vi "Move LabVIEW File.vi"(8 "error in (no error)":errorcluster, 10 "New Path":path, 11 "Existing Path":path) -> (0 "error out":errorcluster)   [LabVIEW 2016, in "SLL Scripting.lvlib"]
uses:
  SLL Scripting.lvlib
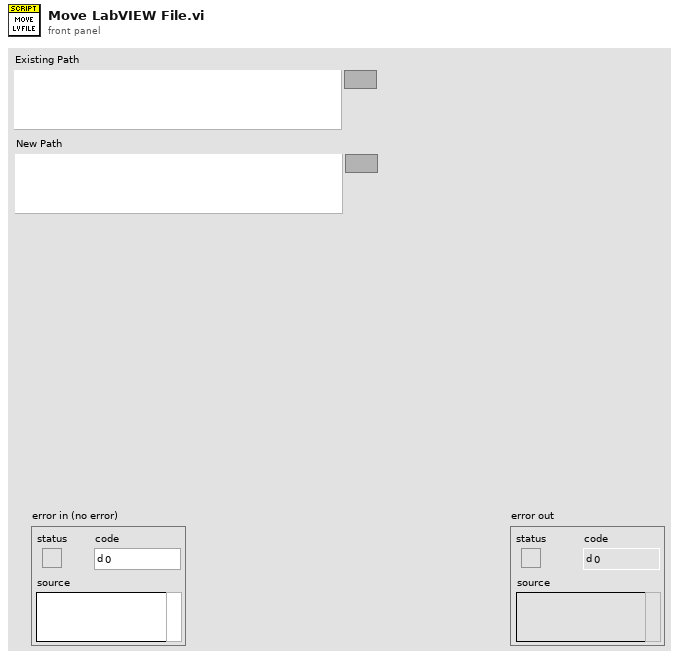
[diagram p1: front panel]
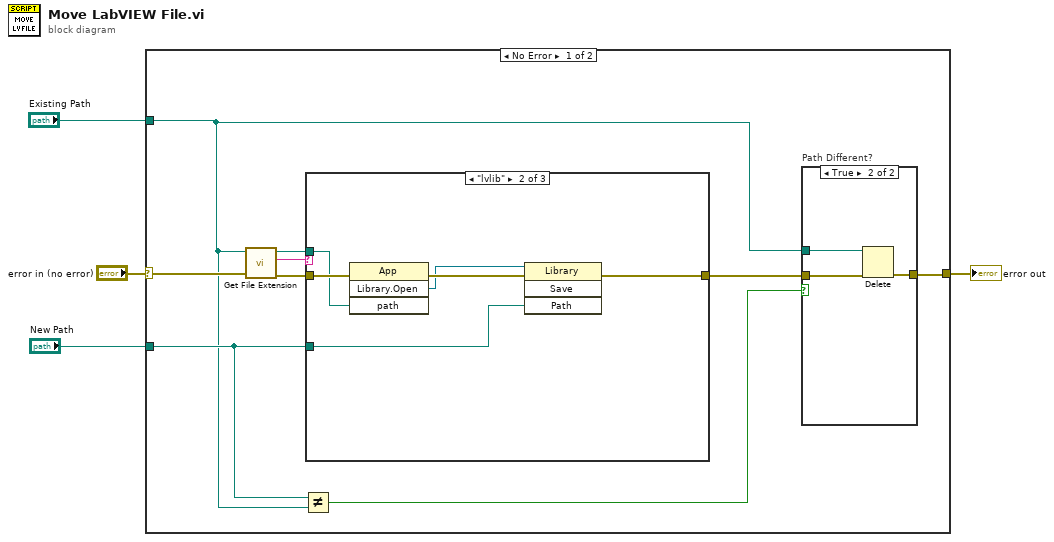
[diagram p0: block diagram]
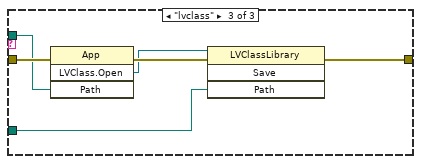
[diagram p4: hidden frame]
diagram:
  n1 = case shown="No Error" "error in (no error)" {
    selector: "error in (no error)" -> [w10 w31]
    tunnel: [w8 w31] -> w3
    tunnel: "New Path" -> [w9 _]
    tunnel: "Existing Path" -> [w6 _]
    frame No Error {
      n2 = call <vilib>:"Get File Extension.vi"("error in (no error)"=w10, "file"=w6) -> ("error out"=w13:errorcluster, "lowercase file extension"=w12:string, "dup file"=w11:path)  [unwired: 5 in, 2 out]
      n3 = Not Equal?(x=w9, y=w6) -> (x != y?=w5:bool)
      n4 = case shown="\"lvlib\"" w12 {
        tunnel: w13 -> [w18 w24 w30]
        tunnel: [w18 w21 w27] -> w7
        tunnel: w11 -> [_ w22 w28]
        tunnel: w9 -> [_ w19 w25]
        frame Default {
        }
        frame "lvlib" {
          n5 = invoke class="App" method="Library.Open"(error in=w24, "path"=w22) -> (error out=w23:errorcluster, "Open Library"=w20:refnum<vi>)  [unwired: 2 in, 2 out]
          n6 = invoke class="Library" method="Save"(reference=w20, error in=w23, "Path"=w19) -> (error out=w21:errorcluster)  [unwired: 1 in, 3 out]
        }
        frame "lvclass" {
          n7 = invoke class="App" method="LVClass.Open"(error in=w30, "Path"=w28) -> (error out=w29:errorcluster, "LVClass.Open"=w26:refnum<vi>)  [unwired: 2 in, 2 out]
          n8 = invoke class="LVClassLibrary" method="Save"(reference=w26, error in=w29, "Path"=w25) -> (error out=w27:errorcluster)  [unwired: 1 in, 3 out]
        }
      }
      n9 = case "Path Different?" shown="True" w5 {
        tunnel: [w14 w17] -> w8
        tunnel: w7 -> [w14 w16]
        tunnel: w6 -> [_ w15]
        frame False {
        }
        frame True {
          n10 = Delete(path (use dialog)=w15, error in=w16) -> (error out=w17:errorcluster)  [unwired: 3 in, 2 out]
        }
      }
    }
    frame Error {
    }
  }
  "error out" <- w3
